vi "health_fiber.vi"(0 "fiberSerial":T1={"port1"="COM1", "port2"="COM1", "timeout"=1000, "baud"=9600, "dataBits"=8, "stopBits"=10, "flowControl"=0, "parity"=0, "termChar"=FALSE, "checkSum"=FALSE, "fiber1On"=FALSE, "fiber2On"=FALSE} {"stopBits" items=["1.0"=10, "1.5"=15, "2.0"=20]; "parity" items=["None", "Odd", "Even", "Mark", "Space"]; "flowControl" items=["None"=0, "XON/XOFF"=1, "RTS/CTS"=2, "DTR/DSR"=4]}, 1 "Address":string, 2 "Channel":string, 3 "Error In":errorcluster) -> (7 "Value":dbl, 8 "Retries":i32, 10 "Error Out":errorcluster)   [LabVIEW 2018]
doc: "The Basic Serial Read and Write example performs a Serial Port Read, a Serial Port Write, or a combination of these actions. The user selects the actions (read or write) on the front panel. If both are selected, the VI will write the data first, read data, and then close the VISA session that is opened to the port. This VI will wait until the specified number of bytes is received at the port. Only the number of bytes specified will be read.\n\nINSTRUCTIONS:\n1) Select the serial resource and configuration parameters (baud rate, data bits, parity, stop bits, flow control).\n2) Select the operations to be performed. \n3) Connect the serial port to your device. If no device is available, perform a loopback test by doing one of the following. Short pins 2 and 3 on a RS-232 cable or short pin 4 to pin 8 and pin 5 to pin 9 on a RS-485/422 cable. \n4) Run the VI to see the data read. (The \"read string\" will match the \"string to write\" if a loopback test was performed.)\n\nNote: The parameters set for the serial port must match the parameters of the connected instrument or device. In this example, the bytes to read parameter specifies the number of bytes that the serial port reads. If there were more bytes at the port than the number specified in bytes to read, those bytes would not be read. Also, if you specify to read more bytes than the number of bytes actually read, you might receive a timeout error message.\n\nOn the block diagram, the Configure Serial Port VI sets the configuration parameters. The front panel displays the controls used to configure the basic parameters, such as baud rate, data bits, and parity. Constants configure the other parameters the user probably does not need set. After the VISA Configure Serial Port VI opens the VISA session and configures the port, the VI passes the VISA resource name to other VIs that perform operations on that VISA resource. The VISA Write function sends a command to the serial device and the VISA Read function returns data based on the command. The VISA Close function then closes the reference to the serial device. It is important to close the reference; otherwise communication through with that port through protocols other than VISA might not be possible."
uses:
  <vilib>/Instr/_visa.llb/VISA Configure Serial Port (Instr).vi
panel:
  out "Fiber Data":dbl[](array[numeric])
  # "RF / Fiber Optic Modem Data"
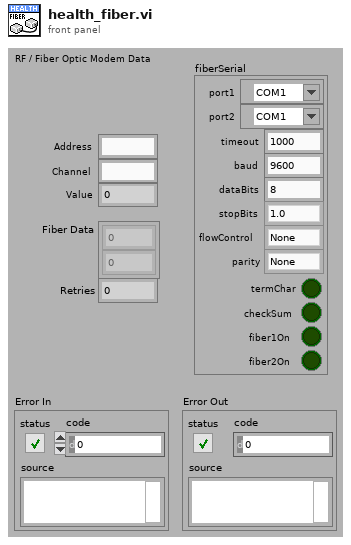
[diagram p1: front panel]
types:
  T1 = cluster{"port1":refnum<visa-resource-name>, "port2":refnum<visa-resource-name>, "timeout":u32, "baud":u32, "dataBits":u16, "stopBits":u16, "flowControl":u16, "parity":u16, "termChar":bool, "checkSum":bool, "fiber1On":bool, "fiber2On":bool}
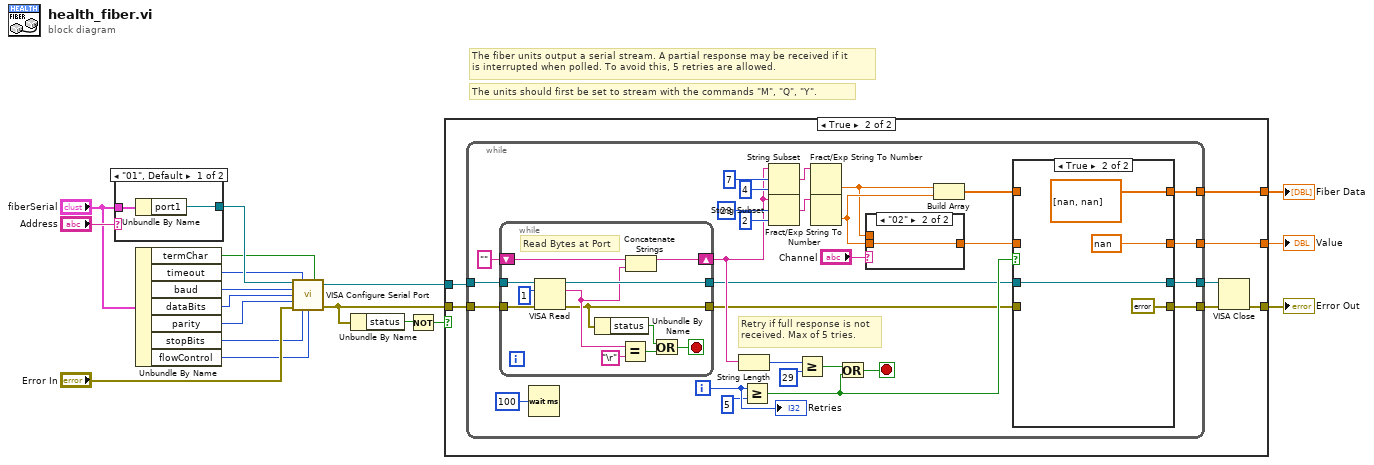
[diagram p0: block diagram]
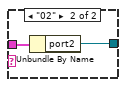
[diagram p2: hidden frame]
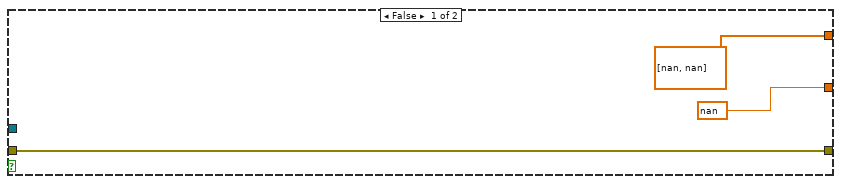
[diagram p3: hidden frame]
diagram:
  # "The units should first be set to stream with the commands \"M\", \"Q\", \"Y\"."
  # "The fiber units output a serial stream. A partial response may be received if it\nis interrupted when polled. To avoid this, 5 retries are allowed."
  n1 = case shown="\"01\", Default" "Address" {
    tunnel: "fiberSerial" -> [w20 w22]
    tunnel: [w19 w21] -> w10
    frame "01", Default {
      n2 = Unbundle By Name(w20) -> ("port1"=w19:refnum<visa-resource-name>)
    }
    frame "02" {
      n3 = Unbundle By Name(w22) -> ("port2"=w21:refnum<visa-resource-name>)
    }
  }
  n4 = Unbundle By Name("fiberSerial") -> ("termChar"=w8:bool, "timeout"=w7:u32, "baud"=w6:u32, "dataBits"=w5:u16, "parity"=w4:u16, "stopBits"=w3:u16, "flowControl"=w2:u16)
  n5 = call-poly "VISA Configure Serial Port"("VISA resource name"=w10, "timeout (10sec)"=w7, "Enable Termination\nChar (T)"=w8, "baud rate (9600)"=w6, "data bits (8)"=w5, "parity (0:none)"=w4, "error in (no error)"="Error In", "stop bits (10: 1 bit)"=w3, "flow control (0:none)"=w2) -> ("VISA resource name out"=w18:refnum<visa-resource-name>, "error out"=w17:errorcluster)  [unwired: 5 in]
  n6 = Unbundle By Name(w17) -> ("status"=w15:bool)
  n7 = Not(x=w15) -> (.not. x?=w16:bool)
  n8 = case shown="True" w16 {
    tunnel: w18 -> [_ w32]
    tunnel: w17 -> [w25 w31]
    tunnel: [w25 w29] -> w13
    tunnel: [dbl[] [nan, nan] w26] -> w14
    tunnel: [nan w27] -> w1
    frame False {
    }
    frame True {
      n9 = while {
        tunnel: [w36] -> w30
        tunnel: w32 -> [w60]
        tunnel: w31 -> [w59]
        tunnel: [w34] -> w28
        tunnel: [w40] -> w27
        tunnel: [w38] -> w26
        i -> [w56]
        stop <- w53 stop-if-true
        # "Retry if full response is not\nreceived. Max of 5 tries."
        n10 = while {
          tunnel: [w72] -> w35
          tunnel: [w83] -> w33
          tunnel: w60 -> [w81]
          shift-right: [w78] -> w42
          shift-left: "" ("read buffer") -> [w79]
          tunnel: w59 -> [w73]
          stop <- w76 stop-if-true
          # "Read Bytes at Port"
          n11 = VISA Read(VISA resource name=w81, byte count=u32 1, error in (no error)=w73) -> (VISA resource name out=w83:refnum<visa-resource-name>, read buffer=w77:string, error out=w72:errorcluster)  [unwired: 1 out]
          n12 = Unbundle By Name(w72) -> ("status"=w74:bool)
          n13 = Equal?(x=w77, y="\r") -> (x = y?=w75:bool)
          n14 = Concatenate Strings(w79, w77) -> (w78:string)
          n15 = Or(x=w74, y=w75) -> (x .or. y?=w76:bool)
        }
        n16 = Wait (ms)(milliseconds to wait=u32 100) -> ()  [unwired: 1 out]
        n17 = String Length(string=w42) -> (length=w57:i32)
        n18 = Greater Or Equal?(x=w56, y=5) -> (x >= y?=w41:bool)
        n19 = String Subset(string=w42, offset (0)=7, length (rest)=4 ("length (rest)")) -> (substring=w47:string)
        n20 = String Subset(string=w42, offset (0)=23, length (rest)=2 ("length (rest)")) -> (substring=w46:string)
        n21 = Greater Or Equal?(x=w57, y=29) -> (x >= y?=w54:bool)
        n22 = Fract/Exp String To Number(string=w47) -> (number=w43:dbl)  [unwired: 3 in, 1 out]
        n23 = Fract/Exp String To Number(string=w46) -> (number=w44:dbl)  [unwired: 3 in, 1 out]
        n24 = Or(x=w54, y=w41) -> (x .or. y?=w53:bool)
        n25 = case shown="\"02\"" "Channel" {
          tunnel: [w70 w71] -> w39
          tunnel: w44 -> [_ w71]
          tunnel: w43 -> [w70 _]
          frame "01", Default {
          }
          frame "02" {
          }
        }
        n26 = Build Array(w43, w44) -> (w37:dbl[])
        n27 = case shown="True" w41 {
          tunnel: [w65 nan] -> w40
          tunnel: w39 -> [w65 _]
          tunnel: [w64 dbl[] [nan, nan]] -> w38
          tunnel: w37 -> [w64 _]
          tunnel: [w62 errorcluster {"status"=TRUE, "code"=-2905, "source"="VISA Read in health_fiber.vi. Max number of retried exceeded."} ("error out")] -> w36
          tunnel: w35 -> [w62 _]
          tunnel: [w63 w67] -> w34
          tunnel: w33 -> [w63 w67]
          frame False {
          }
          frame True {
          }
        }
        "Retries" <- w56
      }
      n28 = VISA Close(VISA resource name=w28, error in (no error)=w30) -> (error out=w29:errorcluster)
    }
  }
  "Fiber Data" <- w14
  "Error Out" <- w13
  "Value" <- w1
